vi "Set OP and Post OP Measurements.vi"(8 "error in (no error)":errorcluster, 11 "Servo to Power Out in":refnum<class "Servo to Power Out.lvclass">) -> (0 "error out":errorcluster, 3 "Servo to Power Out out":refnum<class "Servo to Power Out.lvclass">)   [LabVIEW 2018, in "Servo to Power Out.lvlib" / "Servo to Power Out.lvclass"]
uses:
  Servo to Power Out.lvclass
  Plugins/Measurements/Servo MSMT.lvlibp/Servo MSMT.lvclass
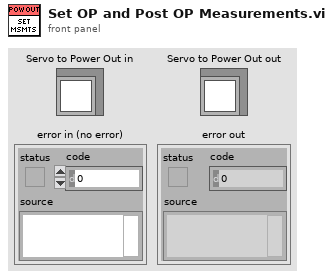
[diagram p1: front panel]
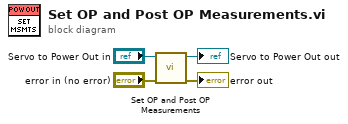
[diagram p0: block diagram]
diagram:
  n1 = call-parent "Set OP and Post OP Measurements.vi"("error in (no error)"="error in (no error)", "Servo MSMT in"="Servo to Power Out in") -> ("error out"=→"error out":errorcluster, "Servo MSMT out"=→"Servo to Power Out out":refnum<class "Servo to Power Out.lvclass">)  [unwired: 8 in]
